vi "FakeToggle (SubVI).vi"(6 "Stage position":refnum<vi>, 7 "Motion direction":string, 8 "error in (no error)":errorcluster, 9 "Axis Speeds":T2={"X [mm/s]"=10.0, "Y [mm/s]"=10.0, "Z [mm/s]"=10.0}, 10 "Jog step size":T1={"X [mm]"=0.001, "Y [mm]"=0.001, "Z [mm]"=0.001}, 11 "Original position":cluster{"X":dbl, "Y":dbl, "Z":dbl}) -> (0 "error out":errorcluster, 2 "Current stage position [mm]":cluster{"X":dbl, "Y":dbl, "Z":dbl})   [LabVIEW 2016]
uses:
  <vilib>/regexp/Match Regular Expression.xnode
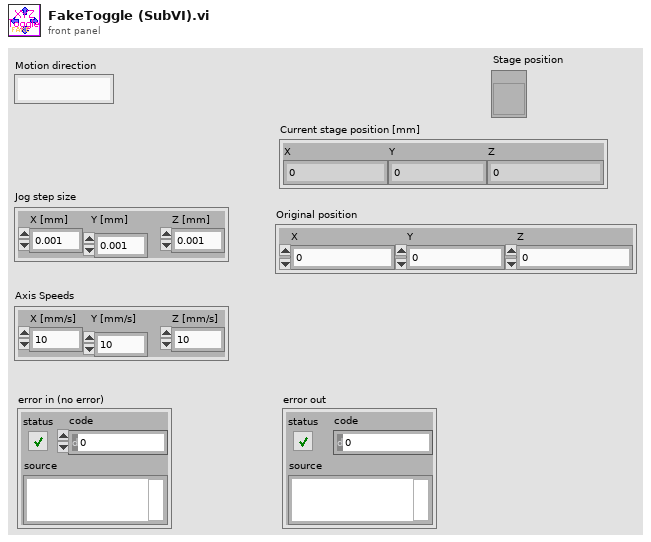
[diagram p1: front panel]
types:
  T1 = cluster{"X [mm]":dbl, "Y [mm]":dbl, "Z [mm]":dbl}
  T2 = cluster{"X [mm/s]":dbl, "Y [mm/s]":dbl, "Z [mm/s]":dbl}
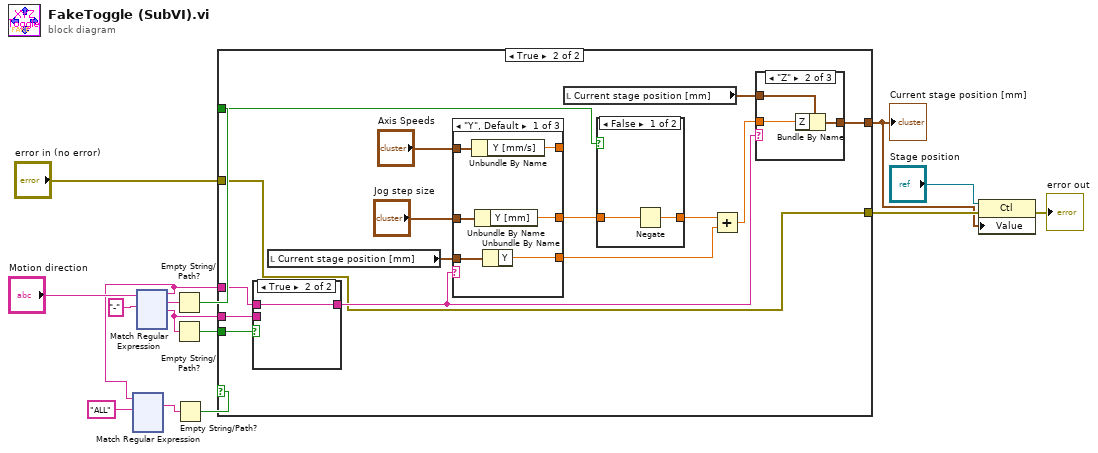
[diagram p0: block diagram]
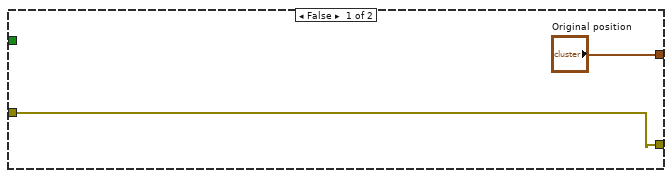
[diagram p2: hidden frame]
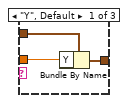
[diagram p3: hidden frame]
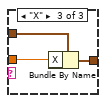
[diagram p4: hidden frame]
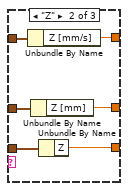
[diagram p7: hidden frame]
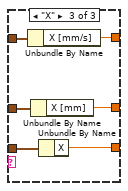
[diagram p8: hidden frame]
diagram:
  n1 = xnode "Match Regular Expression"("input string"="Motion direction", "regular expression"="-") -> ("before match"=w2:string, "whole match"=w10:string, "after match"=w13:string)  [unwired: 4 in, 2 out]
  n2 = xnode "Match Regular Expression"("input string"=w2, "regular expression"="ALL") -> ("whole match"=w3:string)  [unwired: 4 in, 4 out]
  n3 = Empty String/Path?(string/path=w10) -> (empty?=w11:bool)
  n4 = Empty String/Path?(string/path=w13) -> (empty?=w12:bool)
  n5 = Empty String/Path?(string/path=w3) -> (empty?=w4:bool)
  n6 = case shown="True" w4 {
    tunnel: [w16 w18] -> w15
    tunnel: w2 -> [_ w30]
    tunnel: w13 -> [_ w29]
    tunnel: w12 -> [_ w28]
    tunnel: w11 -> [_ w27]
    tunnel: ["Original position" w19] -> w7
    tunnel: "error in (no error)" -> [w16 w18]
    frame False {
    }
    frame True {
      n7 = case shown="True" w28 {
        tunnel: w30 -> [_ w43]
        tunnel: [w42 w43] -> w22
        tunnel: w29 -> [w42 _]
        frame False {
        }
        frame True {
        }
      }
      n8 = local read "Current stage position [mm]"() -> (w25:cluster{"X":dbl, "Y":dbl, "Z":dbl})
      n9 = case shown="\"Y\", Default" w22 {
        tunnel: [w51 w57 w64] -> w26
        tunnel: [w52 w58 w63] -> _
        tunnel: "Jog step size" -> [w50 w56 w62]
        tunnel: "Axis Speeds" -> [w49 w55 w61]
        tunnel: w25 -> [w48 w54 w60]
        tunnel: [w47 w53 w59] -> w23
        frame "Y", Default {
          n10 = Unbundle By Name(w49) -> ("Y [mm/s]"=w52:dbl)
          n11 = Unbundle By Name(w50) -> ("Y [mm]"=w51:dbl)
          n12 = Unbundle By Name(w48) -> ("Y"=w47:dbl)
        }
        frame "Z" {
          n13 = Unbundle By Name(w55) -> ("Z [mm/s]"=w58:dbl)
          n14 = Unbundle By Name(w56) -> ("Z [mm]"=w57:dbl)
          n15 = Unbundle By Name(w54) -> ("Z"=w53:dbl)
        }
        frame "X" {
          n16 = Unbundle By Name(w61) -> ("X [mm/s]"=w63:dbl)
          n17 = Unbundle By Name(w62) -> ("X [mm]"=w64:dbl)
          n18 = Unbundle By Name(w60) -> ("X"=w59:dbl)
        }
      }
      n19 = local read "Current stage position [mm]"() -> (w21:cluster{"X":dbl, "Y":dbl, "Z":dbl})
      n20 = case shown="False" w27 {
        tunnel: w26 -> [w44 w46]
        tunnel: [w45 w46] -> w24
        frame False {
          n21 = Negate(x=w44) -> (-x=w45:dbl)
        }
        frame True {
        }
      }
      n22 = Add(x=w24, y=w23) -> (x+y=w20:dbl)
      n23 = case shown="\"Z\"" w22 {
        tunnel: w21 -> [w35 w36 w41]
        tunnel: w20 -> [w34 w38 w40]
        tunnel: [w33 w37 w39] -> w19
        frame "Y", Default {
          n24 = Bundle By Name(cluster=w35, "Y"=w34) -> (w33:cluster{"X":dbl, "Y":dbl, "Z":dbl})
        }
        frame "Z" {
          n25 = Bundle By Name(cluster=w36, "Z"=w38) -> (w37:cluster{"X":dbl, "Y":dbl, "Z":dbl})
        }
        frame "X" {
          n26 = Bundle By Name(cluster=w41, "X"=w40) -> (w39:cluster{"X":dbl, "Y":dbl, "Z":dbl})
        }
      }
    }
  }
  "Current stage position [mm]" <- w7
  n27 = property class="Ctl"(reference="Stage position", error in=w15, "Value"=w7) -> (error out=→"error out":errorcluster)  [unwired: 1 out]
